vi "Cargo Ship Outake.vi"   [LabVIEW 2018]
uses:
  Cargo Intake Global.vi
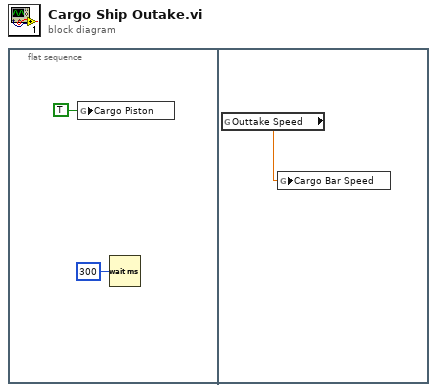
[diagram p0: block diagram]
diagram:
  n1 = flat-sequence {
    frame #0 {
      n2 = global write "Cargo Intake Global.vi" "Cargo Piston"(TRUE ("Cargo Piston")) -> ()
      n3 = Wait (ms)(milliseconds to wait=u32 300) -> ()  [unwired: 1 out]
    }
    frame #1 {
      n4 = global read "Cargo Intake Global.vi" "Outtake Speed"() -> (w3:dbl)
      n5 = global write "Cargo Intake Global.vi" "Cargo Bar Speed"(w3) -> ()
    }
  }
